vi "LIDAR Slave Globals.vi"() -> ()   [LabVIEW 2015]
panel:
  in  "Mode":bool
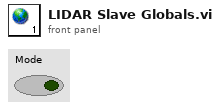
[diagram p1: front panel]
diagram:
